vi "onHttpPatch (File).vi"(8 "error in":errorcluster, 10 "httpRequest":refnum<class "httpRequest.lvclass">, 11 "advanced-http-client in":refnum<class "advanced-http-client.lvclass">) -> (0 "error out":errorcluster, 2 "httpResponse":refnum<class "httpResponse.lvclass">, 3 "advanced-http-client out":refnum<class "advanced-http-client.lvclass">)   [LabVIEW 2020, in "HttpClient.NiAdvanced.lvlib" / "advanced-http-client.lvclass"]
uses:
  advanced-http-client.lvclass
  http-client-pkg/httpRequest/httpRequest.lvclass
  http-client-pkg/httpResponse/httpResponse.lvclass
  advanced-http-client.lvclass/advanced-http-client.ctl
  http-client-pkg/httpRequest/httpRequest.lvclass/httpRequest.ctl
  http-client-pkg/httpRequest/Read output file.vi
  http-client-pkg/httpRequest/Read url.vi
  http-client-pkg/httpRequest/Read buffer.vi
  http-client-pkg/httpRequest/Read timeout.vi
  <vilib>/NI/Advanced HTTP Client/PATCH (File).vi
  <vilib>/NI/Advanced HTTP Client/Session.lvclass
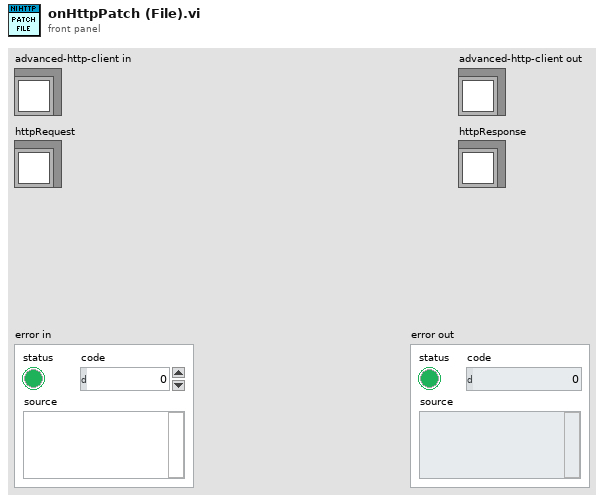
[diagram p1: front panel]
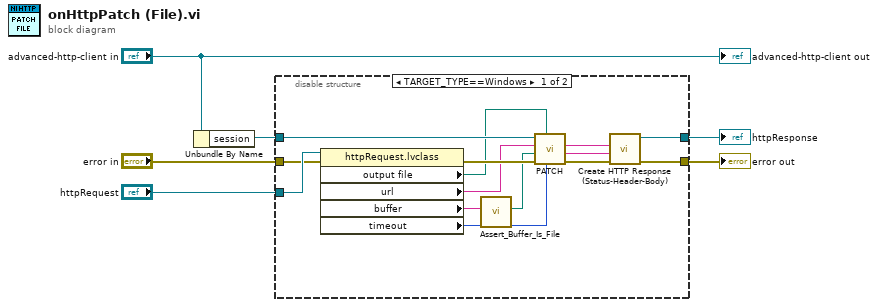
[diagram p0: block diagram]
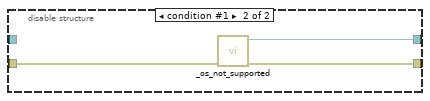
[diagram p2: hidden frame]
diagram:
  n1 = Unbundle By Name("advanced-http-client in") -> ("session"=w3:refnum<class "Session.lvclass">)
  n2 = disable-structure shown="TARGET_TYPE==Windows" {
    disable-tunnel: "error in" -> [w17 w23]
    disable-tunnel: [w10 w22] -> w4
    disable-tunnel: w3 -> [w20 _]
    disable-tunnel: "httpRequest" -> [w19 _]
    disable-tunnel: [w9 w21] -> w1
    frame condition #0 (active) {
      n3 = property class="httpRequest.lvclass"(reference=w19, error in=w17) -> (error out=w18:errorcluster, "output file"=w15:path, "url"=w14:string, "buffer"=w13:string, "timeout"=w16:i32)  [unwired: 1 out]
      n4 = call "Assert_Buffer_Is_File.vi"("buffer"=w13) -> ("File"=w12:path)  [unwired: 9 in, 1 out]
      n5 = call-poly <vilib>:"PATCH.vi"("timeout"=w16, "output file"=w15, "error in"=w18, "file"=w12, "url"=w14, "session in"=w20) -> ("error out"=w11:errorcluster, "body"=w8:string, "headers"=w7:string)  [unwired: 1 in, 2 out]
      n6 = call "Create HTTP Response (Status-Header-Body).vi"("error in"=w11, "body"=w8, "Headers w/ status line(s)"=w7) -> ("error out"=w10:errorcluster, "httpResponse out"=w9:refnum<class "httpResponse.lvclass">)  [unwired: 7 in]
    }
    frame condition #1 {
      n7 = call "_os_not_supported.vi"("error in (no error)"=w23) -> ("error out"=w22:errorcluster, "httpResponse"=w21:refnum<class "httpResponse.lvclass">)  [unwired: 9 in]
    }
  }
  "error out" <- w4
  "httpResponse" <- w1
  "advanced-http-client out" <- "advanced-http-client in"
